vi "TIFFStream Close.vi"(8 "error in (no error)":errorcluster, 10 "Image data reference":refnum<data-value>, 11 "File data":T1) -> (0 "error out":errorcluster)   [LabVIEW 2015]
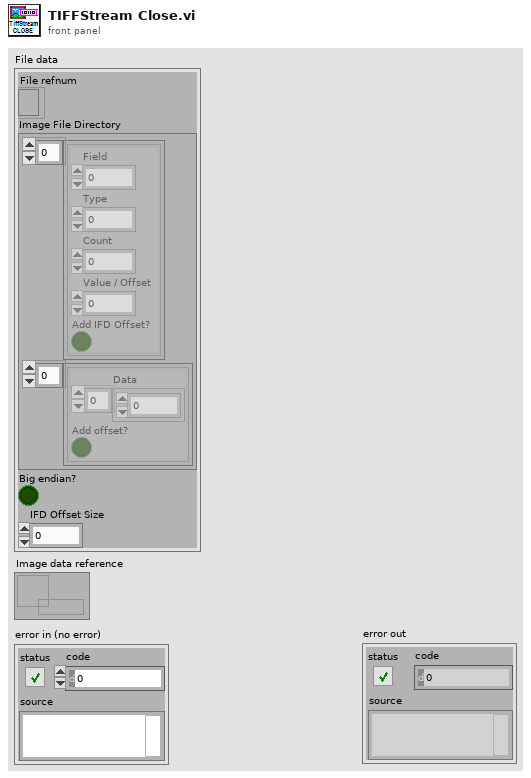
[diagram p1: front panel]
types:
  T1 = cluster{"File refnum":refnum<file>, "Image File Directory":cluster{cluster{"Field":u16, "Type":u16, "Count":u32, "Value / Offset":u32, "Add IFD Offset?":bool}[], cluster{"Data":u32[], "Add offset?":bool}[]}, "Big endian?":bool, "IFD Offset Size":u32}
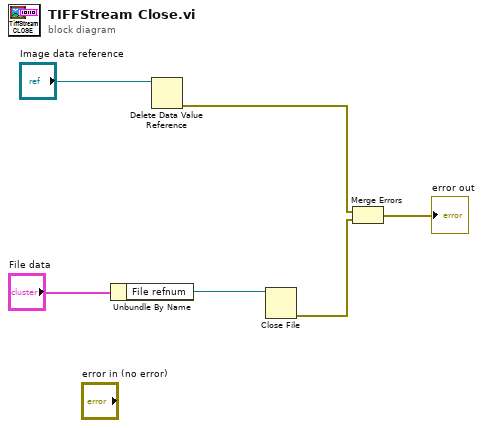
[diagram p0: block diagram]
diagram:
  n1 = Unbundle By Name("File data") -> ("File refnum"=w4:refnum<file>)
  n2 = Delete Data Value Reference(data value reference="Image data reference") -> (error out=w3:errorcluster)  [unwired: 1 in, 1 out]
  n3 = Close File(refnum=w4) -> (error out=w2:errorcluster)  [unwired: 1 in, 1 out]
  n4 = Merge Errors(w3, w2) -> (→"error out":errorcluster)
